vi "Restrict X Domain of Graph_retrieve program.vi"(2 "XY Graph":cluster{"Y":dbl[], "Y":dbl[]}[](array[cluster]), 3 "X Scale.Range:Maximum":dbl, 4 "X Scale.Range:Minimum":dbl) -> (0 "Cluster 2":cluster{"Y":dbl[], "Y":dbl[]}, 1 "Cluster":cluster{dbl[], dbl[]})   [LabVIEW 2016]
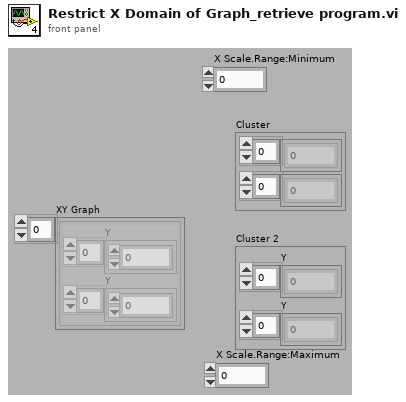
[diagram p1: front panel]
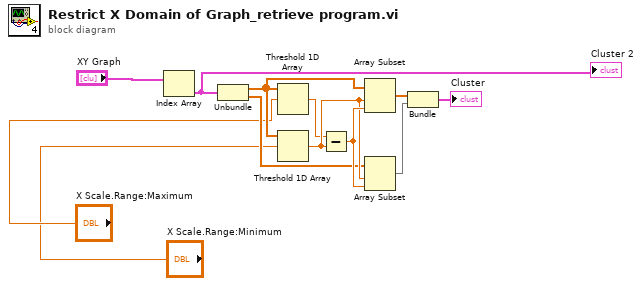
[diagram p0: block diagram]
diagram:
  n1 = Index Array(array="XY Graph") -> (element=w2:cluster{"Y":dbl[], "Y":dbl[]})  [unwired: 1 in]
  "Cluster 2" <- w2
  n2 = Unbundle(w2) -> ("Y"=w6:dbl[], "Y"=w7:dbl[])
  n3 = Threshold 1D Array(2:"X Scale.Range:Maximum", 3:w6) -> (0:w5:dbl)  [unwired: 1 out]
  n4 = Threshold 1D Array(2:"X Scale.Range:Minimum", 3:w6) -> (0:w8:dbl)  [unwired: 1 out]
  n5 = Subtract(x=w5, y=w8) -> (x-y=w9:dbl)
  n6 = Array Subset(array=w6, index=w8, length=w9) -> (w11:dbl[])
  n7 = Array Subset(array=w7, index=w8, length=w9) -> (w10:dbl[])
  n8 = Bundle(w11, w10) -> (→"Cluster":cluster{dbl[], dbl[]})  [unwired: 1 out]
